vi "Set Low Press.vi"(0 "reference in":refnum<class "Stand.lvclass">, 5 "AI index":T1 items=["AI 0 Cooling Station Level", "AI 1 Cooling Station Temp", "AI 2 Oil Supply Level", "AI 3 Oil Supply Temp", "AI 4 ", "AI 5 Pressure Haskel", "AI 6 Pressure DUT", "AI 7 Pressure Chamber", "AI 8 Pressure Air inlet", "AI 9 Pressure Air outlet", "AI 10 Pressure Messure Line"], 11 "error in (no error)":errorcluster) -> (15 "error out":errorcluster)   [LabVIEW 2019, in "Stand.lvclass"]
uses:
  Stand.lvclass
  FPGA_API_class/FPGA API.lvclass
  AI_class/AI.lvclass
  Device_class/Device.lvclass
  D:/GIT H4000/H4000/src/Device_class/Device.lvclass
  FPGA/TypeDef/AI index.ctl
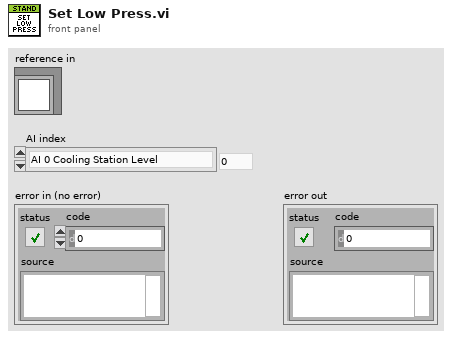
[diagram p1: front panel]
types:
  T1 = typedef "AI index.ctl" = u8
  T2 = typedef "AI_Data.ctl" = cluster{"Stat Data":T3, "OutOfRangeMax":bool, "OutOfRangeMin":bool, "HIHI":bool, "HI":bool, "LO":bool, "LOLO":bool, "DATA N":T4, "DATA PERIOD":T4, "UPPER TH":dbl, "LOWER TH":dbl}
  T3 = typedef "AI Statistics Data.ctl" = cluster{"raw mean":dbl, "scl mean":dbl, "raw mean 1Hz":dbl, "scl mean 1Hz":dbl}
  T4 = typedef "DATA Oscill.ctl" = cluster{"SUM":dbl, "COUNTER":dbl, "MAX CURR":dbl, "MIN CURR":dbl, "AVR":dbl, "MAX":dbl, "MIN":dbl, "DELTA AVR":dbl, "DELTA MAX":dbl, "DELTA MIN":dbl, "PERIOD":dbl}
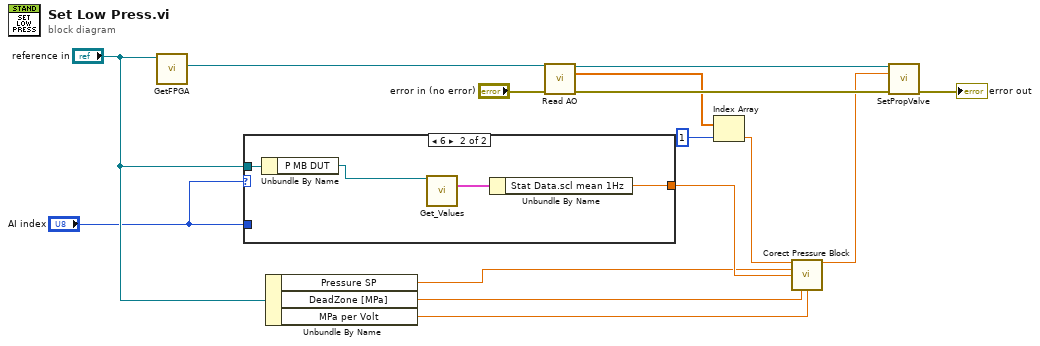
[diagram p0: block diagram]
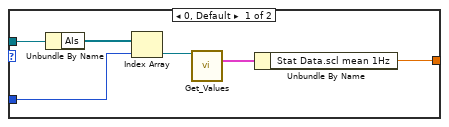
[diagram p2: hidden frame]
diagram:
  n1 = call "GetFPGA.vi"("Device in"="reference in") -> ("FPGA API.lvclass"=w15:refnum<class "FPGA API.lvclass">)  [unwired: 10 in]
  n2 = case shown="6" "AI index" {
    tunnel: "reference in" -> [w21 w25]
    tunnel: [w20 w24] -> w11
    tunnel: "AI index" -> [w17 _]
    frame 0, Default {
      n3 = Unbundle By Name(w21) -> ("AIs"=w16:refnum<class "AI.lvclass">[])
      n4 = Index Array(array=w16, index=w17) -> (element=w18:refnum<class "AI.lvclass">)
      n5 = call "Get_Values.vi"("reference in"=w18) -> ("Data"=w19:T2)  [unwired: 14 in]
      n6 = Unbundle By Name(w19) -> ("Stat Data.scl mean 1Hz"=w20:dbl)
    }
    frame 6 {
      n7 = Unbundle By Name(w25) -> ("P MB DUT"=w22:refnum<class "AI.lvclass">)
      n8 = call "Get_Values.vi"("reference in"=w22) -> ("Data"=w23:T2)  [unwired: 14 in]
      n9 = Unbundle By Name(w23) -> ("Stat Data.scl mean 1Hz"=w24:dbl)
    }
  }
  n10 = Unbundle By Name("reference in") -> ("Pressure SP"=w3:dbl, "DeadZone [MPa]"=w12:dbl, "MPa per Volt"=w13:dbl)
  n11 = call-dynamic "Read AO.vi"("FPGA API in"=w15, "error in (no error)"="error in (no error)") -> ("FPGA API out"=w8:refnum<class "FPGA API.lvclass">, "AO"=w5:dbl[], "error out"=w9:errorcluster)  [unwired: 11 in]
  n12 = Index Array(array=w5, index=1) -> (element=w6:dbl)
  n13 = call "Corect Pressure Block.vi"("U in"=w6, "SP [MPa]"=w3, "PV [MPa]"=w11, "delta"=w12, "MPa per Volt"=w13) -> ("U out"=w7:dbl)  [unwired: 10 in]
  n14 = call-dynamic "SetPropValve.vi"("FPGA API in"=w8, "Do"=w7, "error in (no error)"=w9) -> ("error out"=→"error out":errorcluster)  [unwired: 10 in, 2 out]
